vi "Host_PulsehistogramSimple3GHz.vi"() -> ()   [LabVIEW 2012]
uses:
  <vilib>/FPGAPlugInAG/PXIe-7962R/niLvFpga_Open_PXIe-7962R.vi
  <vilib>/rvi/interface/common/dynamic/niFpgaDynamicAddResources.vi
  <vilib>/Utility/error.llb/Error Cluster From Error Code.vi
  <vilib>/rvi/errors/niLvFpgaAdjustHostInterfaceError.vi
  <vilib>/FPGAPlugInAG/Dynamic/niLvFpga_Close_Dynamic.vi
  <vilib>/rvi/interface/nirviOpenFPGA/nirviOpenFPGA.xnode
  FPGA Bitfiles/PulsehistogramSimple3GHz_NI5771.lvbitx
  <vilib>/rvi/interface/nirviReadWriteControl/nirviReadWriteControl.xnode
  <vilib>/rvi/interface/nirviMethod/nirviMethod.xnode
  <vilib>/rvi/interface/nirviCloseFPGA/nirviCloseFPGA.xnode
  NiFpgaLv.dll
  <vilib>/rvi/interface/Simulation/niFpgaSimulationCallBeginRW.vi
  <vilib>/Analysis/NI_AALPro.lvlib
  <vilib>/FPGAPlugInAG/Dynamic/niLvFpga_ReadFifo_Dynamic.vi
  <vilib>/rvi/errors/niLvFpgaMergeErrorWithErrorCode.vi
panel:
  out "Waveform Graph":u8[](graph)
  in  "AI Channel":enum16{"AI 0", "AI 1"}(ring)
  out "TIS Configuration Error":bool
  out "Loop counter":i32
  out "ToHostU64FIFO Overflow":bool
  out "error out":errorcluster
  out "Histogram Graph":T1(graph)
  out "Configured?":bool
  # "3 GHz TIS mode"
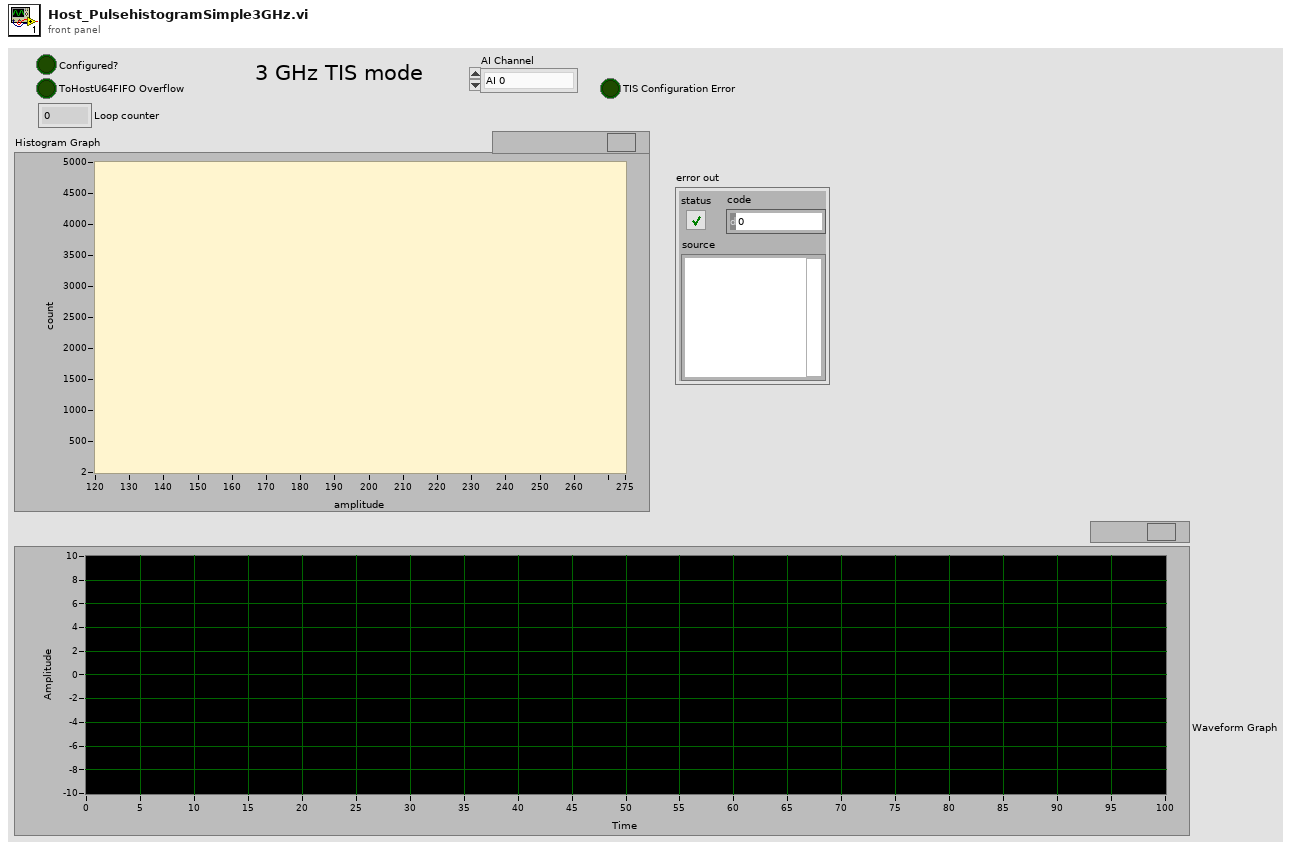
[diagram p1: front panel]
types:
  T1 = cluster{"X Values":dbl[], "Histogram: h(x)":i32[]}
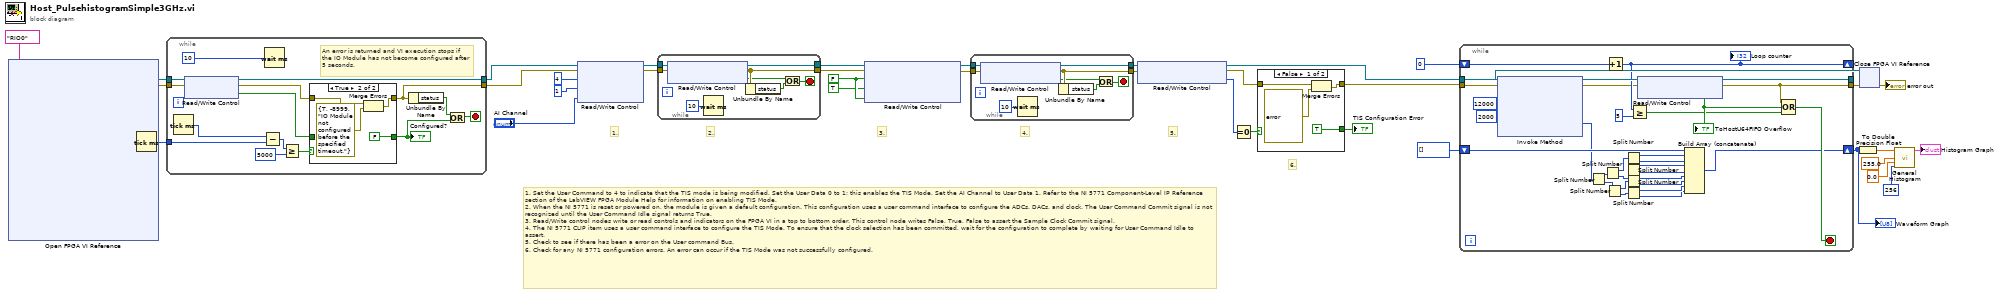
[diagram p0: block diagram]
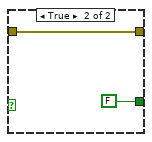
[diagram p2: hidden frame]
diagram:
  w18 = FALSE ("Sample Clock Commit")
  # "5."
  # "6."
  # "4."
  # "3."
  # "2."
  # "1."
  # "1. Set the User Command to 4 to indicate that the TIS mode is being modified. Set the User Data 0 to 1; this enables the TIS Mode. Set the AI Channel to User Data 1. Refer to the NI 5771 Component-Level IP Reference section of the LabVIEW FPGA Module Help for information on enabling TIS Mode.\n2. When the NI 5771 is reset or powered on, the module is given a default configuration. This configuration uses a user command interface to configure the ADCs, DACs, and clock. The User Command Commit signal is not recognized until the User Command Idle signal returns True.\n3. Read/Write control nodes write or read controls and indicators on the FPGA VI in a top to bottom order. This control node writes False, True, False to assert the Sample Clock Commit signal.\n4. The NI 5771 CLIP item uses a user command interface to configure the TIS Mode. To ensure that the clock selection has been committed, wait for the configuration to complete by waiting for User Command Idle to assert.\n5. Check to see if there has been a error on the User command Bus.\n6. Check for any NI 5771 configuration errors. An error can occur if the TIS Mode was not successfully configured."
  n1 = xnode "Open FPGA VI Reference"("resource name"=tag "RIO0") -> ("FPGA VI Reference Out"=w24:refnum<k20>, "error out"=w25:errorcluster)  [unwired: 1 in]
  n2 = Tick Count (ms)() -> (millisecond timer value=w35:u32)
  n3 = while {
    tunnel: w25 -> [w44]
    tunnel: [w48] -> w5
    tunnel: [w40] -> w4
    tunnel: w24 -> [w43]
    tunnel: w35 -> [w38]
    stop <- w46 stop-if-true
    # "An error is returned and VI execution stops if the IO Module has not become configured after 5 seconds."
    n4 = Tick Count (ms)() -> (millisecond timer value=w39:u32)
    n5 = xnode "Read/Write Control"("FPGA VI Reference In"=w43, "error in"=w44) -> ("FPGA VI Reference Out"=w40:refnum<k20>, "error out"=w41:errorcluster, "Configured?"=w42:bool)
    n6 = Subtract(x=w39, y=w38) -> (x-y=w37:u32)
    n7 = Wait (ms)(milliseconds to wait=u32 10) -> ()  [unwired: 1 out]
    n8 = Greater Or Equal?(x=w37, y=u32 5000) -> (x >= y?=w49:bool)
    n9 = case shown="True" w49 {
      tunnel: [w53 FALSE ("Configured?")] -> w45
      tunnel: w42 -> [w53 _]
      tunnel: [w52 w56] -> w48
      tunnel: w41 -> [w52 w54]
      frame False {
      }
      frame True {
        n10 = Merge Errors(w54, errorcluster {"status"=TRUE, "code"=-8999, "source"="IO Module not configured before the specified timeout."} ("error in")) -> (w56:errorcluster)
      }
    }
    "Configured?" <- w45
    n11 = Unbundle By Name(w48) -> ("status"=w47:bool)
    n12 = Or(x=w47, y=w45) -> (x .or. y?=w46:bool)
  }
  n13 = xnode "Read/Write Control"("FPGA VI Reference In"=w4, "error in"=w5, "User Command"=u8 4, "User Data 0"=u8 1, "User Data 1"="AI Channel") -> ("FPGA VI Reference Out"=w22:refnum<k20>, "error out"=w21:errorcluster)
  n14 = while {
    tunnel: w22 -> [w61]
    tunnel: w21 -> [w62]
    tunnel: [w59] -> w19
    tunnel: [w60] -> w20
    stop <- w63 stop-if-true
    n15 = xnode "Read/Write Control"("FPGA VI Reference In"=w61, "error in"=w62) -> ("FPGA VI Reference Out"=w60:refnum<k20>, "error out"=w59:errorcluster, "User Command Idle"=w58:bool)
    n16 = Wait (ms)(milliseconds to wait=u32 10) -> ()  [unwired: 1 out]
    n17 = Unbundle By Name(w59) -> ("status"=w64:bool)
    n18 = Or(x=w58, y=w64) -> (x .or. y?=w63:bool)
  }
  n19 = xnode "Read/Write Control"("FPGA VI Reference In"=w20, "error in"=w19, "User Command Commit"=w18, "User Command Commit"=TRUE ("Sample Clock Commit"), "User Command Commit"=w18) -> ("FPGA VI Reference Out"=w16:refnum<k20>, "error out"=w15:errorcluster)
  n20 = while {
    tunnel: w16 -> [w69]
    tunnel: w15 -> [w70]
    tunnel: [w67] -> w14
    tunnel: [w68] -> w13
    stop <- w71 stop-if-true
    n21 = xnode "Read/Write Control"("FPGA VI Reference In"=w69, "error in"=w70) -> ("FPGA VI Reference Out"=w68:refnum<k20>, "error out"=w67:errorcluster, "User Command Idle"=w66:bool)
    n22 = Wait (ms)(milliseconds to wait=u32 10) -> ()  [unwired: 1 out]
    n23 = Unbundle By Name(w67) -> ("status"=w72:bool)
    n24 = Or(x=w66, y=w72) -> (x .or. y?=w71:bool)
  }
  n25 = xnode "Read/Write Control"("FPGA VI Reference In"=w13, "error in"=w14) -> ("FPGA VI Reference Out"=w2:refnum<k20>, "error out"=w11:errorcluster, "User Command Status"=w9:u8)
  n26 = Equal To 0?(x=w9) -> (x = 0?=w8:bool)
  n27 = case shown="False" w8 {
    tunnel: [w77 w79] -> w3
    tunnel: w11 -> [w76 w79]
    tunnel: [TRUE ("Configured?") FALSE ("Configured?")] -> w10
    frame False {
      n28 = Merge Errors(w76, errorcluster {"status"=TRUE, "code"=-8998, "source"="IO Module clock not configured correctly. Please ensure that the desired clock meets the required specifications."} ("error in")) -> (w77:errorcluster)
    }
    frame True {
    }
  }
  "TIS Configuration Error" <- w10
  n29 = while {
    tunnel: w3 -> [w85]
    tunnel: w2 -> [w86]
    tunnel: [w109] -> w34
    tunnel: [w110] -> w33
    shift-right: [w88] -> w1
    shift-left: u8[] [] -> [w87]
    shift-right: [w105] -> _
    shift-left: 0 -> [w106]
    stop <- w107 stop-if-true
    n30 = xnode "Invoke Method"("FPGA VI Reference In"=w86, "error in"=w85, "Number of Elements"=u32 12000, "Timeout (ms)"=2000) -> ("FPGA VI Reference Out"=w80:refnum<k20>, "error out"=w81:errorcluster, "Data"=w82:u64[])  [unwired: 1 out]
    n31 = Split Number(x=w82) -> (hi(x)=w102:u32[], lo(x)=w101:u32[])
    n32 = Split Number(x=w102) -> (hi(x)=w100:u16[], lo(x)=w99:u16[])
    n33 = Split Number(x=w101) -> (hi(x)=w98:u16[], lo(x)=w97:u16[])
    n34 = Increment(x=w106) -> (x+1=w105:i32)
    "Loop counter" <- w105
    n35 = Split Number(x=w100) -> (hi(x)=w96:u8[], lo(x)=w95:u8[])
    n36 = Split Number(x=w99) -> (hi(x)=w94:u8[], lo(x)=w93:u8[])
    n37 = Split Number(x=w98) -> (hi(x)=w92:u8[], lo(x)=w91:u8[])
    n38 = Split Number(x=w97) -> (hi(x)=w90:u8[], lo(x)=w89:u8[])
    n39 = Greater Or Equal?(x=w105, y=5) -> (x >= y?=w103:bool)
    n40 = xnode "Read/Write Control"("FPGA VI Reference In"=w80, "error in"=w81) -> ("FPGA VI Reference Out"=w110:refnum<k20>, "error out"=w109:errorcluster, "ToHostFIFO Overflow"=w108:bool)
    "ToHostU64FIFO Overflow" <- w108
    n41 = Build Array (concatenate)(w87, w96, w95, w94, w93, w92, w91, w90, w89) -> (w88:u8[])
    n42 = Compound Arithmetic op=OR(w109, w108, w103) -> (w107:bool)
  }
  "Waveform Graph" <- w1
  n43 = To Double Precision Float(number=w1) -> (double precision float=w28:dbl[])
  n44 = xnode "Close FPGA VI Reference"("FPGA VI Reference In"=w33, "error in"=w34) -> ("error out"=→"error out":errorcluster)
  n45 = call <vilib>:"General Histogram.vi"("X"=w28, "max"=255.0, "min"=0.0, "# bins"=256) -> ("Histogram Graph"=→"Histogram Graph":T1)  [unwired: 7 in, 4 out]
